vi "Set default values.vi"(8 "error in (no error)":errorcluster, 11 "device data model in":refnum<class "ELAN Data Model.lvclass">) -> (0 "error out":errorcluster, 3 "device data model out":refnum<class "ELAN Data Model.lvclass">)   [LabVIEW 2021, in "ELAN Data Model.lvclass"]
doc: "This VI ensures that the data model has at least 65,535 values of every type. This is required for certain modbus function codes."
uses:
  ELAN Data Model.lvclass
  ELAN Data Model.lvclass/ELAN Data Model.ctl
  Type Definitions/Value full.ctl
  Data Unit/ELAN PC Data Unit/Elan units.ctl
  Data Unit/ELAN PC Data Unit/Elan measured variable.ctl
  Data Unit/ELAN PC Data Unit/Elan channel state.ctl
  Type Definitions/Data Model.ctl
  Data Unit/ELAN PC Data Unit/ELAN PDU.lvclass
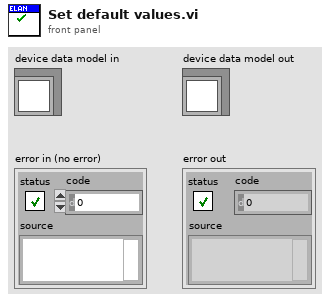
[diagram p1: front panel]
types:
  T1 = typedef "ELAN Data Model.lvclass/Value full.ctl" = cluster{"Value":cluster{"Value":sgl, "units":T2, "component":T3}, "channel state":T4, "collective state":errorcluster}
  T2 = typedef "ELAN PDU.lvclass/Elan units.ctl" = enum16{"Invalid", "no dimension", "ppm", "ppb", "vpm", "ppm C1", "ppm C3", "ppm C6", "mg C/m3", "mg/m3", "%", "% vol", "% of measuring range", "% saturation", "%/°C", "%/K", "% weight", "mV/pH", "mV/mbar", "nA/mbar", "S/m", "S/cm", "mS/m", "mS/cm", "ìS/m", "ìS/cm", "S", "min", "H", "Pa", "MA", "uV", "MV", "V", "mbar", "hPa", "Ml/min", "kOhm", "MOhm", "S1", "°C", "Hz", "pH", "ug/l", "mg/l", "l/min", "uA", "mg/dm3", "kPa", "kOhm*cm", "MOhm*cm", "°", "1/min", "1/m", "g/m3", "g/l", "% Vol C"}
  T3 = typedef "ELAN PDU.lvclass/Elan measured variable.ctl" = enum16{"Invalid", "no component", "CO", "CO2", "CH4 (Methan)", "C6H14 (Hexan)", "SO2", "NO", "NO2", "CHClF2 (R22)", "C3H8 (Propan)", "C4H10 (Butan)", "O2", "C5H12 (Pentan)", "CnHm (THC)", "P (process pressure)", "pH", "T (temperature)", "C2H4 (Ethen)", "C2H2 (Ethin)", "C3H6 (Propen)", "C4H6", "C4H8", "C2H6", "NH3 (Ammoniak)", "N2O", "C6H6 (Benzol)", "SF6", "CH3OH (Methanol)", "C2H5OH (Ethanol)", "CH2Cl2", "C2H4Cl2", "CH3Cl", "C2H4O", "H2O (water vapor)", "G/l (conductivity)", "C", "S", "N", "CF4", "COCl2 (phosgene)", "CHF3 (R23)", "C2F6 (R116)", "------ (self defined component)", "C2H3Cl", "H2 (Hydrogen)", "Ar", "He", "Cl2", "N2"}
  T4 = typedef "ELAN PDU.lvclass/Elan channel state.ctl" = enum16{"Invalid", "Warm-up", "Pause", "Standby", "Measure", "Zero calibration", "Adjust component slope", "Not yet defined1", "Adjust curve dip", "Adjust linearization sensitivity", "Adjust temperature compensation", "Adjust pressure compensation", "Adjust linearization zero", "Not yet defined2", "Autocal", "Adjust phase", "Zero calibration of O2 sensor", "Synchronous zero calibration", "Purging for synchronous zero calibration", "Adjust analog output", "Adjust analog input", "Autocal check"}
  T5 = typedef "ELAN Data Model.lvclass/Data Model.ctl" = cluster{"UTC":u64, "Value":T1[]}
  T6 = typedef "Device Data Model.lvclass/N channel.ctl" = cluster{"N DI channel":i32, "N DO channel":i32, "N AI channel":i32, "N AO channel":i32}
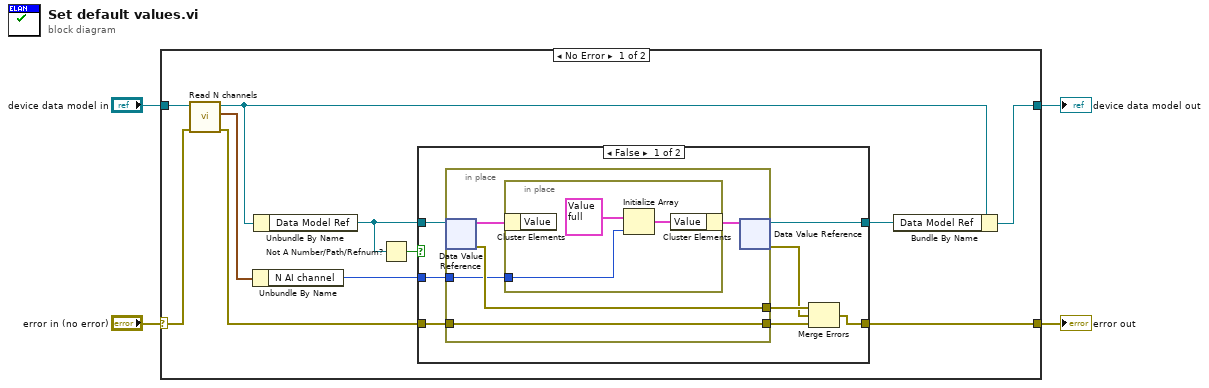
[diagram p0: block diagram]
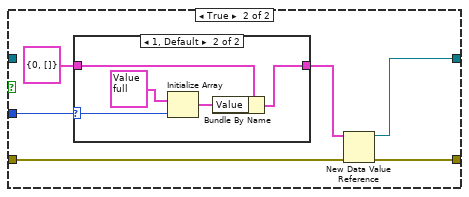
[diagram p2: hidden frame]
diagram:
  n1 = case shown="No Error" "error in (no error)" {
    selector: "error in (no error)" -> [w8 w45]
    tunnel: "device data model in" -> [w10 w44]
    tunnel: [w15 w44] -> w3
    tunnel: [w11 w45] -> w2
    frame No Error {
      n2 = call-dynamic "Read N channels.vi"("error in (no error)"=w8, "device data model in"=w10) -> ("error out"=w7:errorcluster, "N channel"=w6:T6, "device data model out"=w9:refnum<class "ELAN Data Model.lvclass">)  [unwired: 7 in]
      n3 = Unbundle By Name(w6) -> ("N AI channel"=w5:i32)
      n4 = Unbundle By Name(w9) -> ("Data Model Ref"=w13:refnum<data-value>)
      n5 = Not A Number/Path/Refnum?(number/path/refnum=w13) -> (NaN/Path/Refnum?=w12:bool)
      n6 = case shown="False" w12 {
        tunnel: w7 -> [w23 w37]
        tunnel: w13 -> [w22 _]
        tunnel: [w21 w35] -> w14
        tunnel: [w19 w36] -> w11
        tunnel: w5 -> [w16 w32]
        frame False {
          n7 = in-place {
            in-place-border: w23 -> [w27]
            in-place-border: [w28] -> w20
            in-place-border: [w27] -> w17
            in-place-border: w16 -> [w24]
            n8 = in-place-dvr #1(w22) -> (w26:T5, w28:errorcluster)
            n9 = in-place {
              in-place-border: w24 -> [w29]
              n10 = in-place-cluster #2(w26) -> ()  [unwired: 1 out]
              n11 = Initialize Array(T1 {"Value"={"Value"=0.0, "units"=enum."Invalid", "component"=enum."Invalid"}, "channel state"=enum."Invalid", "collective state"={"status"=FALSE, "code"=0, "source"=""}} ("Value full"), w29) -> (w31:T1[])
              n12 = in-place-cluster #2("Value"=w31) -> (w25:T5)
            }
            n13 = in-place-dvr #1(w25) -> (w21:refnum<data-value>, w18:errorcluster)
          }
          n14 = Merge Errors(w20, w18, w17) -> (w19:errorcluster)
        }
        frame True {
          n15 = case shown="1, Default" w32 {
            selector: w32 -> [_ w40]
            tunnel: T5 {"UTC"=0, "Value"=[]} ("Data Model") -> [w38 w43]
            tunnel: [w38 w41] -> w33
            frame 0 {
            }
            frame 1, Default {
              n16 = Initialize Array(T1 {"Value"={"Value"=0.0, "units"=enum."Invalid", "component"=enum."Invalid"}, "channel state"=enum."Invalid", "collective state"={"status"=FALSE, "code"=0, "source"=""}} ("Value full"), w40) -> (w42:T1[])
              n17 = Bundle By Name(cluster=w43, "Value"=w42) -> (w41:T5)
            }
          }
          n18 = New Data Value Reference(data value=w33, error in=w37) -> (data value reference=w35:refnum<data-value>, error out=w36:errorcluster)
        }
      }
      n19 = Bundle By Name(cluster=w9, "Data Model Ref"=w14) -> (w15:refnum<class "ELAN Data Model.lvclass">)
    }
    frame Error {
    }
  }
  "error out" <- w2
  "device data model out" <- w3
